vi "ExtendedKalmanFilter_Correct_OnlyUY.vi"(4 "H_ExtraData":variant, 6 "H":T1, 9 "Y":T2, 10 "U":T2, 11 "in ExtendedKalmanFiilter":T3) -> (0 "Error":bool, 3 "out ExtendedKalmanFiilter":T3)   [LabVIEW 2019, in "Trajectory_Library.lvlib"]
doc: "Correct the state estimate x-hat using the measurements in y.\n \nInputs:\n - inExtendedKalmanFIlter -- filter data cluster\n - u -- Same control input used in the predict step.\n - y -- Measurement vector.\n - h_Func -- A vector-valued function reference of x and u that returns the measurement vector.\n - H_func_extra -- extra data, if any, used by H_Func\n\nReturns:\n - outExtendedKalmanFIlter -- updated filter data cluster\n - error -- If TRUE, an error occured"
uses:
  Trajectory_Library.lvlib
  EXTENDED_KALMAN_FILTER.ctl
  <vilib>/Analysis/Matrix/Datatypes/RealMatrix.ctl
  CALLBACK_FUNC_TYPE.ctl
  <vilib>/Analysis/Matrix/NI_Matrix.lvlib
panel:
  # "<Inputs, 1>"
  # "<Outputs, 1>"
  # "State Estimate <Statess,1>"
  # "<States, States>"
  # "<States, States>"
  # "<Statess,  States>"
  # "<Outputs, Outputs>"
  # "State Estimate <Statess,1>"
  # "<States, States>"
  # "<States, States>"
  # "<Statess,  States>"
  # "<Outputs, Outputs>"
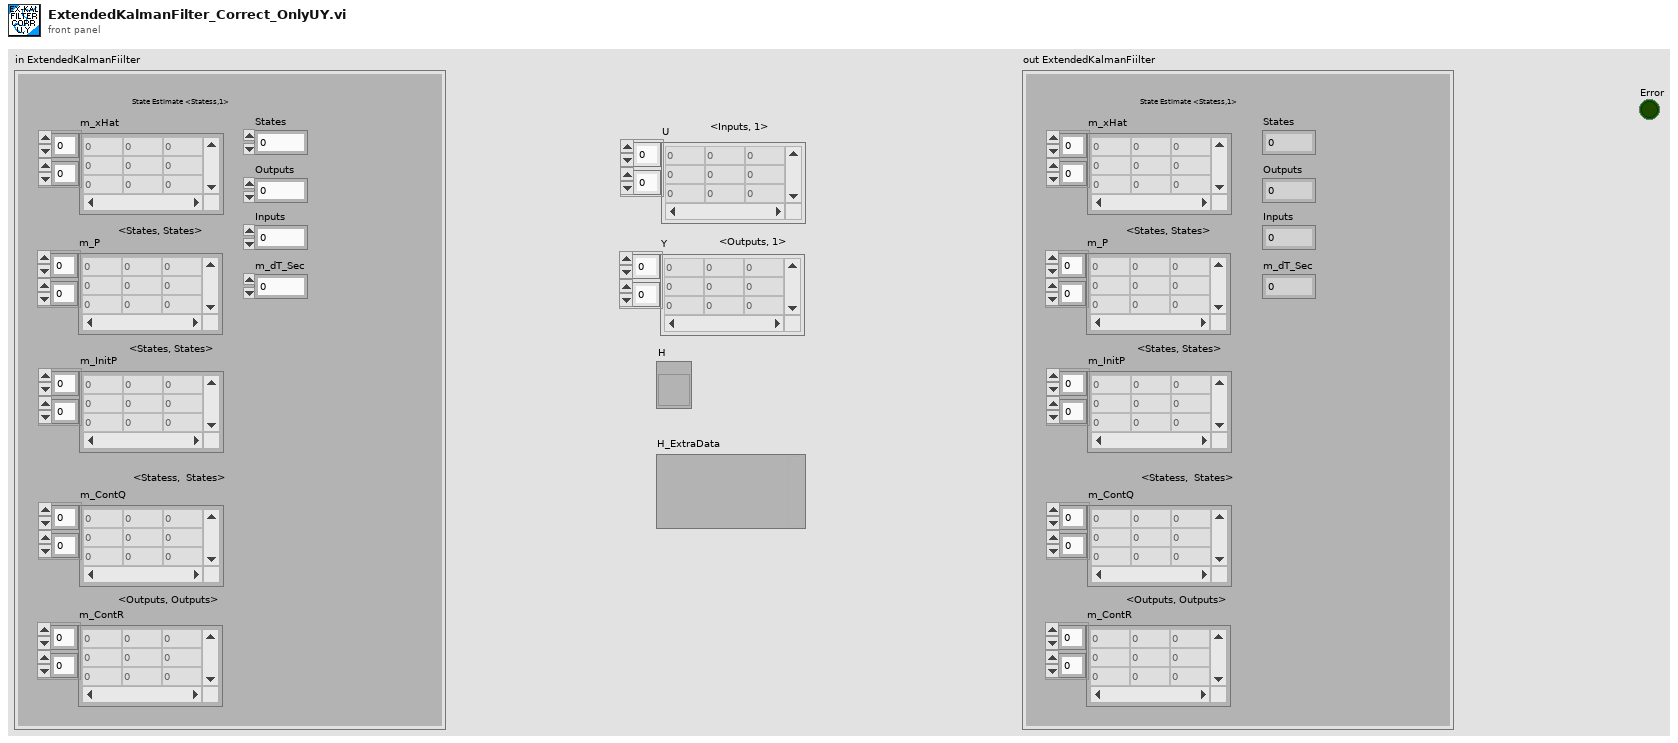
[diagram p1: front panel]
types:
  T1 = typedef "Trajectory_Library.lvlib/CALLBACK_FUNC_TYPE.ctl" = refnum<vi>
  T2 = typedef "NI_Matrix.lvlib/RealMatrix.ctl" = dbl[][]
  T3 = typedef "Trajectory_Library.lvlib/EXTENDED_KALMAN_FILTER.ctl" = cluster{"m_P":T2, "m_xHat":T2, "States":i32, "Outputs":i32, "m_ContR":T2, "m_ContQ":T2, "m_dT_Sec":dbl, "Inputs":i32, "m_InitP":T2}
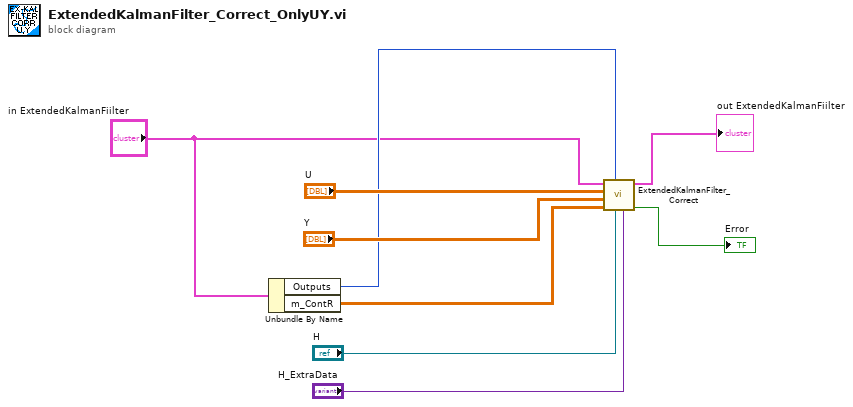
[diagram p0: block diagram]
diagram:
  n1 = Unbundle By Name("in ExtendedKalmanFiilter") -> ("Outputs"=w7:i32, "m_ContR"=w6:T2)
  n2 = call "ExtendedKalmanFilter_Correct.vi"("H_FuncExtra"="H_ExtraData", "H_Func"="H", "Rows"=w7, "R"=w6, "Y"="Y", "U"="U", "in ExtendedKalmanFiilter"="in ExtendedKalmanFiilter") -> ("Error"=→"Error":bool, "out ExtendedKalmanFiilter"=→"out ExtendedKalmanFiilter":T3)  [unwired: 3 in]
